vi "Autotuning PID Offline_JAS.vi"() -> ()   [LabVIEW 2019]
doc: "This example demonstrates how to use the PID Design function to obtain PID parameters based on measured process."
uses:
  <vilib>/Rock Robotics/WPI/ThirdParty/JAS_Junk/TrajLib/PIDController_AtSetpoint.vi
  <vilib>/Rock Robotics/WPI/ThirdParty/JAS_Junk/TrajLib/PIDController_SetPIDF.vi
  <vilib>/Rock Robotics/WPI/ThirdParty/JAS_Junk/TrajLib/PIDController_SetDerivativeFilter.vi
  <vilib>/Rock Robotics/WPI/ThirdParty/JAS_Junk/TrajLib/PIDController_SetIntegratorRange.vi
  <vilib>/Rock Robotics/WPI/ThirdParty/JAS_Junk/TrajLib/PIDController_SetTolerancePandV.vi
  <vilib>/Rock Robotics/WPI/ThirdParty/JAS_Junk/TrajLib/PIDController_DisableContinousInput.vi
  <vilib>/Rock Robotics/WPI/ThirdParty/JAS_Junk/TrajLib/PIDController_EnableContinousInput.vi
  <vilib>/Rock Robotics/WPI/ThirdParty/JAS_Junk/TrajLib/PIDController_Reset.vi
  <vilib>/Rock Robotics/WPI/ThirdParty/JAS_Junk/TrajLib/PIDController_New.vi
  <vilib>/Rock Robotics/WPI/ThirdParty/JAS_Junk/TrajLib/PIDController_SetOutputLimits.vi
  <vilib>/Rock Robotics/WPI/ThirdParty/JAS_Junk/TrajLib/PIDController_NewPeriod.vi
  <vilib>/Rock Robotics/SystemInterfaces/NetworkCommunication/NetComm_UsageReport_report.vi
  <vilib>/Rock Robotics/WPI/ThirdParty/JAS_Junk/TrajLib/Util_LibraryGlobals.vi
  <vilib>/Rock Robotics/WPI/ThirdParty/JAS_Junk/TrajLib/PIDController_AdvCalculate_FF_Sp_Pv.vi
  <vilib>/Rock Robotics/WPI/ThirdParty/JAS_Junk/TrajLib/Trajectory_Library.lvlib
panel:
  in  "Use\nFeedforward":bool
  out "Tuned PID Gains":T1
  in  "CO Offset":dbl=1.0 format="%#_13g"
  out "Tuning Done":bool
  in  "Type of controller":u16(ring)=2 items=["P", "PI", "PID"]
  in  "Control":enum32{"Generic", "Internal Model Control"}(tab)
  in  "Constant Type":T2(ring)
  in  "Multiplicative factor":dbl(slide)=1.0 scale=0.01..100.0
  in  "Tab Control":T3(tab)
  in  "Instructions":string="Overview: This example demonstrates how to use the PID Autotuning Design to obtain PID parameters based on setpoint and process variable collected in another loop.\nInstructions:\n1. Run the VI and wait until the process variable (PV) reaches near setpoint (SP).\n2.  In the PID Autotuning Design section, select the type of algorithm, type of controller and excitation amplitude for the 'open loop step response'. Then, click Autotune to start the process. Select the Identified Plant Parameter tab and see the results from the identification.\n3.  When the tuned PID gains do not change anymore, the identification is done and you have the option to accept by clicking Accept gain, which will transfer the new gain to PID Gains.\n4. Click the Autotune button again to go back to the automatic control state. You can try different options and repeat this process.\n5. Click Stop to stop the VI.\n"
  out "Plant and Test Data":T4
  out "Elapsed Time":dbl format="%13.2f"
  in  "Process parameters":T5={"static gain"=2.5, "lag (s)"=2.5, "deadtime (s)"=0.01, "load"=0.0, "deadband"=0.0, "sensor noise"=0.0, "initial PV"=30.0, "plant noise"=0.0}
  in  "PID \nAuto / Manual":bool=TRUE
  out "CO":dbl(graph)=20.39115328927357
  in  "Accept gain":bool
  in  "Perform PID\nAutoTune":bool
  in  "SP:":dbl(slide)=50.98039215686275 min=0.0 max=0.0 scale=0.0..100.0
  out "CO_":dbl(slide)=20.39115328927357 scale=-100.0..100.0
  out "PV:":dbl(slide)=50.98160323470328 scale=0.0..100.0
  in  "PID Gains":T6={"proportional gain (Kp)"=2.5, "integral time (Ki, /sec)"=4.0, "derivative time (Kd, /sec)"=0.0} {"derivative time (Kd, /sec)" format="%#.6g"; "integral time (Ki, /sec)" format="%#.6g"; "proportional gain (Kp)" format="%#.6g"}
  in  "Sampling Time dt (s)":dbl=0.019999999999999997 min=0.001 step=0.01 format="%#.3p"
  out "SP and PV":cluster{"initial PV":dbl, "SP1:":dbl}(graph)={"initial PV"=50.98160323470328, "SP1:"=50.98039215686275}
  # "Proportional-Integral-Derivative (PID) Controller"
  # "PID Autotuning Design"
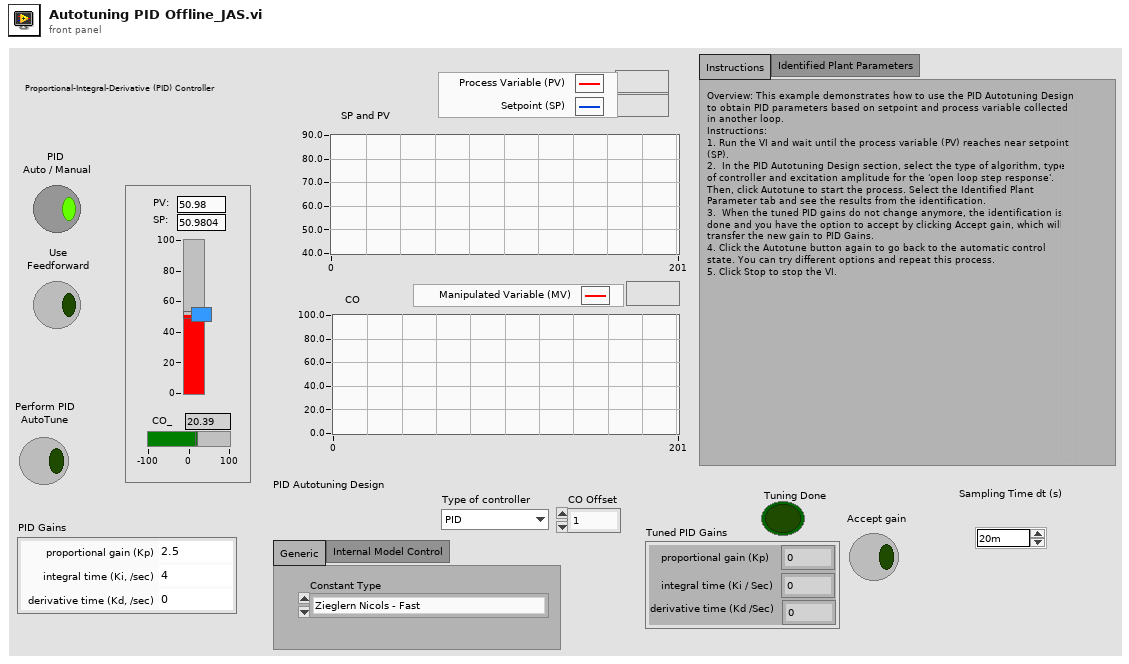
[diagram p1: front panel]
types:
  T1 = cluster{"proportional gain (Kp)":dbl, "integral time (Ki / Sec)":dbl, "derivative time (Kd /Sec)":dbl}
  T2 = enum16{"Zieglern Nicols - Fast", "Ziegler Nicols - Normal", "Ziegler Nicols - Slow", "CHR regulator - 0% overshoot", "CHR regulator - 20% overshoot", "CHR servo - 0 % overshoot", "CHR servo - 20% overshoot"}
  T3 = enum32{"Instructions", "Identified Plant Parameters"}
  T4 = cluster{"Plant Gain (K)":dbl, "Time Constant (T)":dbl, "Dead Time (L)":dbl, "stimulus operating point":dbl, "response operating point":dbl}
  T5 = cluster{"static gain":dbl, "lag (s)":dbl, "deadtime (s)":dbl, "load":dbl, "deadband":dbl, "sensor noise":dbl, "initial PV":dbl, "plant noise":dbl}
  T6 = cluster{"proportional gain (Kp)":dbl, "integral time (Ki, /sec)":dbl, "derivative time (Kd, /sec)":dbl}
  T7 = typedef "Trajectory_Library.lvlib/PID_ADV_LIMITS.ctl" = cluster{"MaxInput":dbl, "MinInput":dbl, "Continuous":bool, "MaxOutput":dbl, "MinOutput":dbl}
  T8 = typedef "Trajectory_Library.lvlib/PID_ADV_TUNING.ctl" = cluster{"Kf":dbl, "Kp":dbl, "Ki":dbl, "Kd":dbl, "MaximumIntegral":dbl, "MinimumIntegral":dbl, "Filter Derivative":bool}
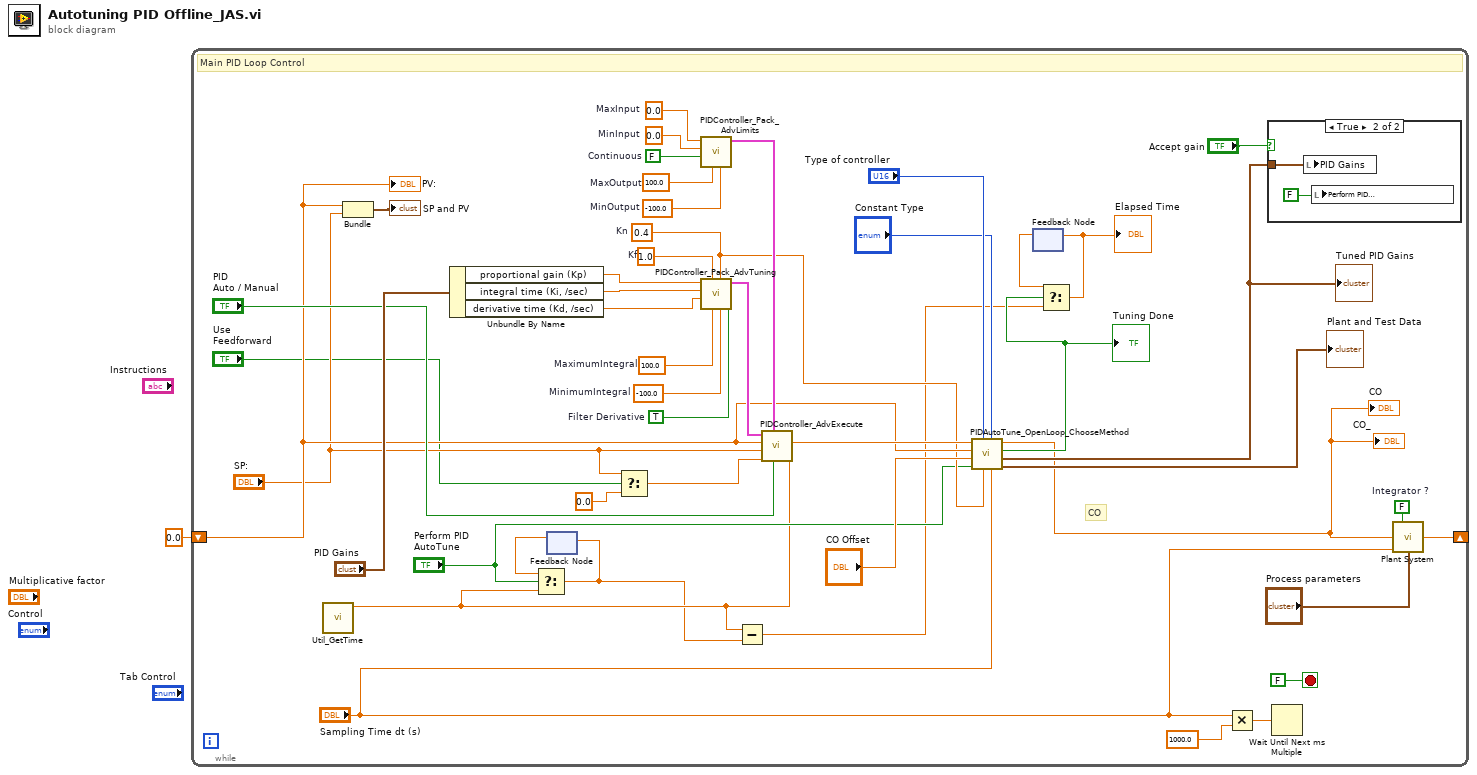
[diagram p0: block diagram]
diagram:
  n1 = while {
    shift-left: 0.0 ("Plant Output") -> [w24]
    shift-right: [w45] -> _
    stop <- FALSE stop-if-true
    w22 = 0.4  # Kn
    w41 = 1.0  # Kf
    w40 = 100.0  # MaximumIntegral
    w39 = -100.0  # MinimumIntegral
    w38 = TRUE  # Filter Derivative
    w36 = 0.0  # MinInput
    w35 = FALSE  # Continuous
    w34 = 100.0  # MaxOutput
    w37 = -100.0  # MinOutput
    w33 = 0.0  # MaxInput
    w46 = FALSE  # Integrator ?
    # "CO"
    # "Main PID Loop Control"
    n2 = call <vilib>:"Util_GetTime.vi"() -> ("FPGA_Time_Seconds"=w13:dbl)  [unwired: 10 in, 1 out]
    n3 = Bundle("Plant Output"=w24, "SP:"="SP:") -> (→"SP and PV":cluster{"Plant Output":dbl, "SP:":dbl})  [unwired: 1 in]
    n4 = Unbundle By Name("PID Gains") -> ("proportional gain (Kp)"=w29:dbl, "integral time (Ki, /sec)"=w28:dbl, "derivative time (Kd, /sec)"=w27:dbl)
    n5 = feedback #1() -> (w14:dbl)  [unwired: 1 in]
    n6 = Select(t=w14, s="Perform PID\nAutoTune", f=w13) -> (s? t:f=w12:dbl)
    n7 = feedback-in #1(w12) -> ()
    n8 = Select(t="SP:", s="Use\nFeedforward", f=0.0) -> (s? t:f=w4:dbl)
    n9 = call <vilib>:"PIDController_Pack_AdvLimits.vi"("MinOutput"=w37, "MaxOutput"=w34, "Continuous"=w35, "MinInput"=w36, "MaxInput"=w33) -> ("Adv PID Limits"=w31:T7)  [unwired: 6 in]
    n10 = call <vilib>:"PIDController_Pack_AdvTuning.vi"("Filter Derivative"=w38, "MinimumIntegral"=w39, "Kn"=w22, "MaximumIntegral"=w40, "Kf"=w41, "Kd"=w27, "Ki"=w28, "Kp"=w29) -> ("Adv PID Tuning"=w32:T8)  [unwired: 3 in]
    n11 = Subtract(x=w13, y=w12) -> (x-y=w10:dbl)
    n12 = call <vilib>:"PIDController_AdvExecute.vi"("Time"=w13, "Auto"="PID \nAuto / Manual", "Adv PID Limits"=w31, "FF-FeedForward"=w4, "SP-SetPoint"="SP:", "PV-Measurement"=w24, "Adv PID Tuning"=w32) -> ("CO-ControlOutput"=w25:dbl)  [unwired: 2 in, 2 out]
    n13 = call <vilib>:"PIDAutoTune_OpenLoop_ChooseMethod.vi"("Sampling Time dt (s)"="Sampling Time dt (s)", "Constant Type"="Constant Type", "Kn"=w22, "Type of Controller"="Type of controller", "Tune"="Perform PID\nAutoTune", "CO Offset"="CO Offset", "Measurement  (PV)"=w24, "Control Output (Co)"=w25) -> ("Plant and Test Data"=→"Plant and Test Data":T4, "New Tuning Parameters"=w17:T1, "Tuning Done"=w11:bool, "Adj CO"=w6:dbl)
    "CO" <- w6
    "CO_" <- w6
    "Tuning Done" <- w11
    "Tuned PID Gains" <- w17
    n14 = feedback #2() -> (w8:dbl)  [unwired: 1 in]
    n15 = Select(t=w8, s=w11, f=w10) -> (s? t:f=w9:dbl)
    "Elapsed Time" <- w9
    n16 = feedback-in #2(w9) -> ()
    n17 = Multiply(x="Sampling Time dt (s)", y=1000.0) -> (x*y=w43:dbl)
    n18 = case shown="True" "Accept gain" {
      tunnel: w17 -> [_ w49]
      frame False {
      }
      frame True {
        n19 = local write "PID Gains"(w49) -> ()
        n20 = local write "Perform PID\nAutoTune"(FALSE ("Autotune")) -> ()
      }
    }
    n21 = Wait Until Next ms Multiple(millisecond multiple=w43) -> ()  [unwired: 1 out]
    n22 = call "Plant System.vi"("Integrator ?"=w46, "Plant Input"=w6, "dt (s)"="Sampling Time dt (s)", "process parameters"="Process parameters") -> ("Plant Output"=w45:dbl)  [unwired: 11 in]
    "PV:" <- w24
  }
